vi "RotationDAQ.vi"(8 "frequency":i32, 9 "pin":i32, 10 "handle":u32, 11 "Tourner?":bool) -> (3 "Succés?":bool)   [LabVIEW 2020]
uses:
  cDaqlib/cDaq.lvlib
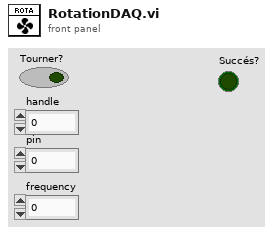
[diagram p1: front panel]
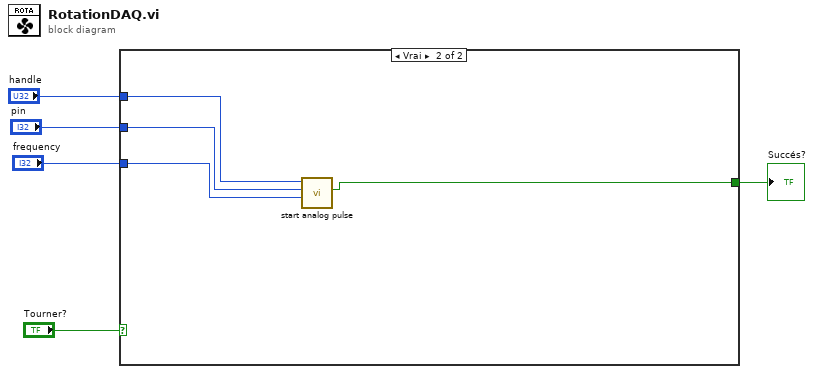
[diagram p0: block diagram]
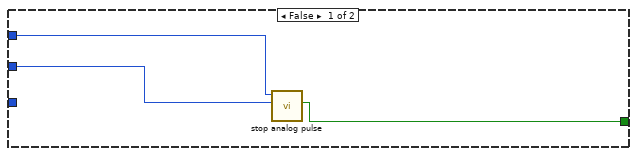
[diagram p2: hidden frame]
diagram:
  n1 = case shown="Vrai" "Tourner?" {
    tunnel: "handle" -> [w8 w12]
    tunnel: "pin" -> [w7 w11]
    tunnel: "frequency" -> [_ w10]
    tunnel: [w6 w9] -> w1
    frame False {
      n2 = call "stop analog pulse .vi"("pin"=w7, "handle"=w8) -> ("function return"=w6:bool)  [unwired: 8 in, 1 out]
    }
    frame True {
      n3 = call "start analog pulse .vi"("frequency"=w10, "pin"=w11, "handle"=w12) -> ("function return"=w9:bool)  [unwired: 7 in, 1 out]
    }
  }
  "Succés?" <- w1
